vi "kernel.vi"(6 "Starting x":dbl, 7 "Array of zeros":dbl[](array[numeric]), 8 "Final x":dbl, 9 "step":dbl, 10 "h":dbl, 11 "current data point":dbl) -> (2 "Points":dbl[](array[numeric]))   [LabVIEW 2009]
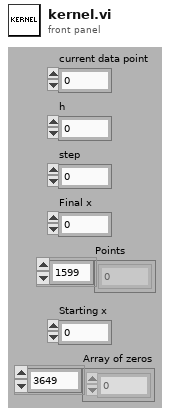
[diagram p1: front panel]
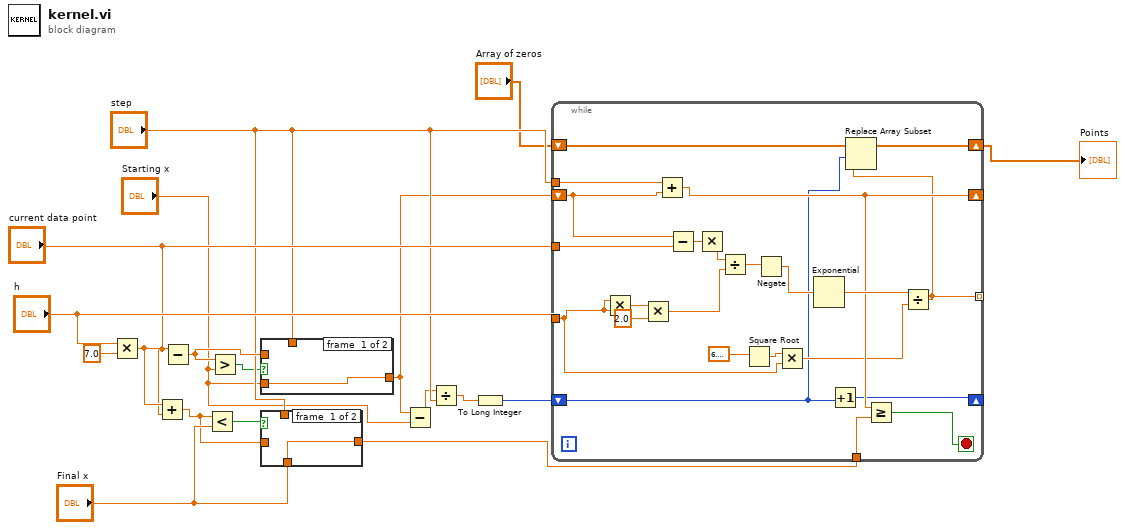
[diagram p0: block diagram]
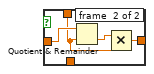
[diagram p2: hidden frame]
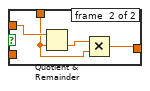
[diagram p3: hidden frame]
diagram:
  n1 = Multiply(x="h", y=7.0) -> (x*y=w16:dbl)
  n2 = Add(x=w16, y="current data point") -> (x+y=w12:dbl)
  n3 = Subtract(x="current data point", y=w16) -> (x-y=w14:dbl)
  n4 = Less?(x=w12, y="Final x") -> (x < y?=w1:bool)
  n5 = Greater?(x=w14, y="Starting x") -> (0:w2:bool)
  n6 = case shown="True" w2 {
    tunnel: [w19 w20] -> w8
    tunnel: "Starting x" -> [w19 _]
    tunnel: w14 -> [_ w23]
    tunnel: "step" -> [_ w21]
    frame #0 {
    }
    frame #1 {
      n7 = Quotient & Remainder(x=w23, y=w21) -> (floor(x/y)=w22:dbl)  [unwired: 1 out]
      n8 = Multiply(x=w22, y=w21) -> (x*y=w20:dbl)
    }
  }
  n9 = case shown="True" w1 {
    tunnel: [w24 w25] -> w11
    tunnel: "Final x" -> [w24 _]
    tunnel: w12 -> [_ w27]
    tunnel: "step" -> [_ w26]
    frame #0 {
    }
    frame #1 {
      n10 = Quotient & Remainder(x=w27, y=w26) -> (floor(x/y)=w28:dbl)  [unwired: 1 out]
      n11 = Multiply(x=w28, y=w26) -> (x*y=w25:dbl)
    }
  }
  n12 = Subtract(x=w8, y="Starting x") -> (x-y=w7:dbl)
  n13 = Divide(x=w7, y="step") -> (x/y=w9:dbl)
  n14 = To Long Integer(number=w9) -> (32bit integer=w4:i32)
  n15 = while {
    shift-right: [w39] -> _
    shift-left: w8 -> [w41]
    tunnel: "current data point" -> [w51]
    tunnel: "h" -> [w34]
    tunnel: "step" -> [w40]
    tunnel: w11 -> [w38]
    shift-right: [w31] -> _
    shift-left: w4 -> [w32]
    shift-right: [w30] -> w3
    shift-left: "Array of zeros" -> [w33]
    tunnel: [w29] -> _ mode=indexing
    stop <- w37 stop-if-true
    n16 = Multiply(x=w34, y=w34) -> (x*y=w49:dbl)
    n17 = Multiply(x=w49, y=2.0) -> (x*y=w47:dbl)
    n18 = Add(x=w40, y=w41) -> (x+y=w39:dbl)
    n19 = Subtract(x=w41, y=w51) -> (x-y=w50:dbl)
    n20 = Multiply(x=w50, y=w50) -> (x*y=w46:dbl)
    n21 = Divide(x=w46, y=w47) -> (x/y=w45:dbl)
    n22 = Square Root(x=6.283185307179586) -> (sqrt(x)=w36:dbl)
    n23 = Negate(x=w45) -> (-x=w44:dbl)
    n24 = Multiply(x=w36, y=w34) -> (x*y=w35:dbl)
    n25 = Exponential(1:w44) -> (0:w43:dbl)
    n26 = Increment(x=w32) -> (x+1=w31:i32)
    n27 = Greater Or Equal?(x=w39, y=w38) -> (x >= y?=w37:bool)
    n28 = Divide(x=w43, y=w35) -> (x/y=w29:dbl)
    n29 = Replace Array Subset(array=w33, new element=w29, index=w32) -> (w30:dbl[])
  }
  "Points" <- w3
